vi "Set Current Position (uSMC).vi"(2 "error in (no error)":errorcluster, 3 "Index":i32, 4 "Visa array in":refnum<visa-resource-name>[](array[refnum])) -> (0 "error out":errorcluster, 1 "Visa array out":refnum<visa-resource-name>[](array[refnum]))   [LabVIEW 2010, in "SignalWriterMH110203USBStepperMotor.lvclass"]
uses:
  SignalWriterMH110203USBStepperMotor.lvclass
  class_data.vi
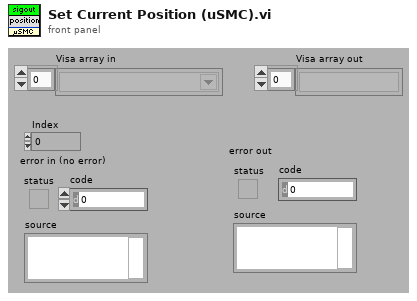
[diagram p1: front panel]
types:
  T1 = cluster{"Cur Pos Units":dbl, "Set Cur Pos units":dbl, "Lo Limit Units":dbl, "Hi Limit Units":dbl, "Cur Pos Ticks":i32, "Set Cur Pos ticks":i32, "Lo Limit Ticks":i32, "Hi Limit Ticks":i32, "Minimal Value":dbl, "Maximal Value":dbl}[]
  T2 = cluster{"Cur Pos Units":dbl, "Set Cur Pos units":dbl, "Lo Limit Units":dbl, "Hi Limit Units":dbl, "Cur Pos Ticks":i32, "Set Cur Pos ticks":i32, "Lo Limit Ticks":i32, "Hi Limit Ticks":i32, "Minimal Value":dbl, "Maximal Value":dbl}
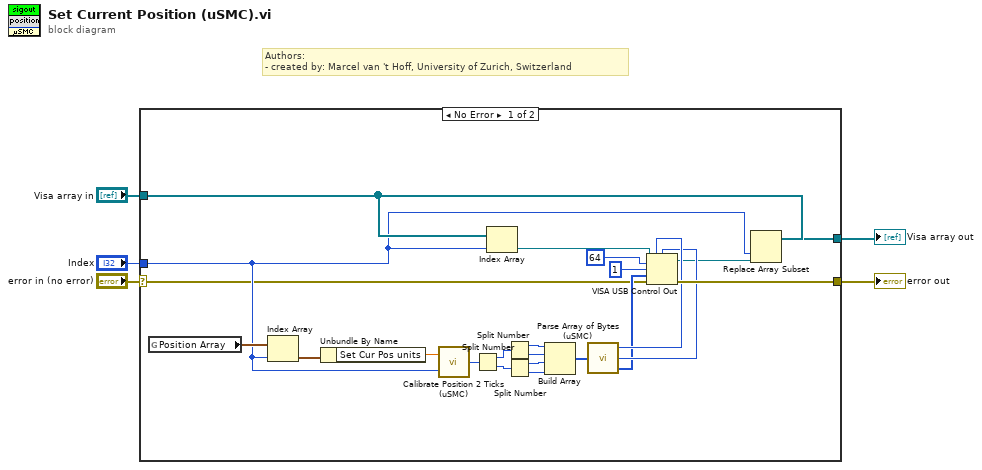
[diagram p0: block diagram]
diagram:
  # "Authors: \n- created by: Marcel van 't Hoff, University of Zurich, Switzerland"
  n1 = case shown="No Error" "error in (no error)" {
    selector: "error in (no error)" -> [w6 w30]
    tunnel: [w26 w30] -> w5
    tunnel: "Visa array in" -> [w13 w29]
    tunnel: [w12 w29] -> w3
    tunnel: "Index" -> [w7 _]
    frame No Error {
      n2 = global read "class_data.vi" "Position Array"() -> (w11:T1)
      n3 = Index Array(array=w11, index=w7) -> (element=w10:T2)
      n4 = Unbundle By Name(w10) -> ("Set Cur Pos units"=w9:dbl)
      n5 = call "Calibrate Position 2 Ticks (uSMC).vi"("array index"=w7, "value"=w9) -> ("value ticks"=w8:i32)
      n6 = Split Number(x=w8) -> (hi(x)=w24:u16, lo(x)=w25:u16)
      n7 = Index Array(array=w13, index=w7) -> (element=w15:refnum<visa-resource-name>)
      n8 = Split Number(x=w24) -> (hi(x)=w23:u8, lo(x)=w22:u8)
      n9 = Split Number(x=w25) -> (hi(x)=w21:u8, lo(x)=w20:u8)
      n10 = Build Array(w23, w22, w21, w20) -> (w19:u8[])
      n11 = call "Parse Array of Bytes (uSMC).vi"("byte array"=w19) -> ("first 2 bytes"=w18:u16, "second 2 bytes"=w17:u16, "array buffer"=w16:u8[])
      n12 = VISA USB Control Out(0:w15, 1:w18, 2:w17, 5:i16 64 ("request type"), 7:i16 1 ("request type"), 9:w16, 11:w6) -> (4:w14:refnum<visa-resource-name>, 15:w26:errorcluster)
      n13 = Replace Array Subset(array=w13, new element=w14, index=w7) -> (w12:refnum<visa-resource-name>[])
    }
    frame Error {
    }
  }
  "error out" <- w5
  "Visa array out" <- w3
